vi "SendMsgByStrType.vi"(8 "error in (no error)":errorcluster, 9 "Data":string, 10 "MSG":string, 11 "MC-ExternClient in":refnum<class "MC-ExternClient.lvclass">) -> (0 "error out":errorcluster, 3 "MC-ExternClient out":refnum<class "MC-ExternClient.lvclass">)   [LabVIEW 2020, in "MC-ExternClient.lvlib" / "MC-ExternClient.lvclass"]
uses:
  MC-ExternClient.lvclass
  C:/Program Files (x86)/National Instruments/LabVIEW 2020/vi.lib/ActorFramework/Actor/Actor.lvclass
  MC-ExternClient.lvclass/MC-ExternClient.ctl
  MC-ExternClientInterface/MC-ExternClientInterface.lvclass
  <vilib>/ActorFramework/Actor/Actor.lvclass/Actor.ctl
  <vilib>/ActorFramework/Message Enqueuer/Message Enqueuer.lvclass/Message Enqueuer.ctl
  <vilib>/ActorFramework/Message Priority Queue/Priority Enqueue.vi
  <vilib>/ActorFramework/Actor/Actor.lvclass
  MailboxManager/MailboxManager Messages/SendMessageToMailbox Msg/SendMessageToMailbox Msg.lvclass
  C:/Users/taylo/Projects/LabVIEW/ActorMailbox/MailboxClient/MailboxClient/MailboxClient.lvclass
  C:/Users/taylo/Projects/LabVIEW/ActorMailbox/MailboxClientInterface/MailboxClientInterface.lvclass
  C:/Users/taylo/Projects/LabVIEW/ActorMailbox/Example/ExternClient/MC-ExternClient/MC-ExternClient/MC-ExternClient.lvclass
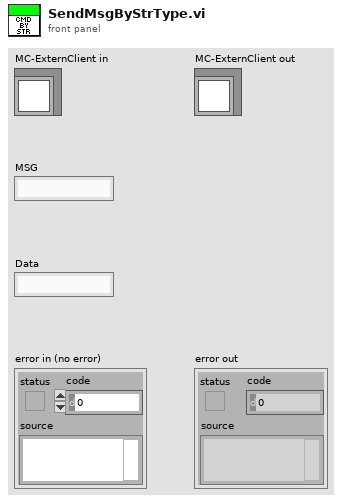
[diagram p1: front panel]
types:
  T1 = map{string, refnum<class "MailBoxMessage.lvclass">}
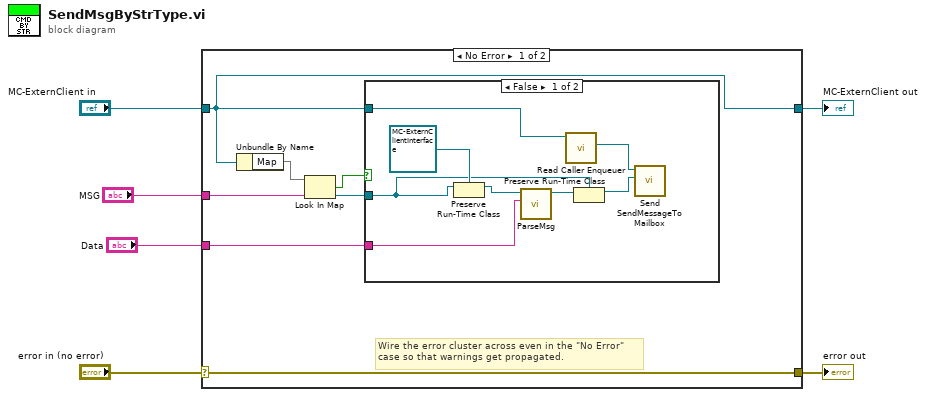
[diagram p0: block diagram]
diagram:
  n1 = case shown="No Error" "error in (no error)" {
    selector: "error in (no error)" -> [w13 w23]
    tunnel: [w13 w23] -> w5
    tunnel: [w9 w22] -> w3
    tunnel: "MC-ExternClient in" -> [w9 w22]
    tunnel: "MSG" -> [w11 _]
    tunnel: "Data" -> [w10 _]
    frame No Error {
      # "Wire the error cluster across even in the \"No Error\"\ncase so that warnings get propagated."
      n2 = Unbundle By Name(w9) -> ("Map"=w12:T1)
      n3 = Look In Map(map=w12, key=w11) -> (key not found?=w7:bool, value=w8:refnum<class "MailBoxMessage.lvclass">)  [unwired: 1 in]
      n4 = case shown="False" w7 {
        tunnel: w10 -> [w19 _]
        tunnel: w9 -> [w18 _]
        tunnel: w8 -> [w16 _]
        frame False {
          n5 = Preserve Run-Time Class(object in=w16, 2:refnum<class "MC-ExternClientInterface.lvclass"> refnum ("MC-ExternClient.lvlib:MC-ExternClientInterface.lvclass")) -> (object out=w20:refnum<class "MC-ExternClientInterface.lvclass">)  [unwired: 1 in, 1 out]
          n6 = call-dynamic "ParseMsg.vi"("ToParse"=w19, "MC-ExternClientInterface in"=w20) -> ("MC-ExternClientInterface out"=w17:refnum<class "MC-ExternClientInterface.lvclass">)  [unwired: 8 in, 1 out]
          n7 = call <vilib>:"Read Caller Enqueuer.vi"("Actor"=w18) -> ("Caller Enqueuer"=w15:refnum<class "Message Enqueuer.lvclass">)  [unwired: 10 in]
          n8 = Preserve Run-Time Class(object in=w17, 2:w16) -> (object out=w14:refnum<class "MailBoxMessage.lvclass">)  [unwired: 1 in, 1 out]
          n9 = call "Send SendMessageToMailbox.vi"("MailBoxMessage"=w14, "Message Enqueuer"=w15) -> ()  [unwired: 8 in, 2 out]
        }
        frame True {
        }
      }
    }
    frame Error {
    }
  }
  "error out" <- w5
  "MC-ExternClient out" <- w3
